vi "Get Information String.vi"(8 "error in (no error)":errorcluster caption="错误输入（无错误）", 11 "PCM PanelSplit.lvclass":refnum<class "PCM PanelSplit.lvclass">) -> (0 "error out":errorcluster caption="错误输出", 2 "Information String out":string, 3 "PCM PanelSplit out":refnum<class "PCM PanelSplit.lvclass"> caption="DNL_LabVIEW Object out")   [LabVIEW 2016, in "PCM PanelSplit.lvclass"]
uses:
  PCM PanelSplit.lvclass
  <vilib>/Analysis/4window.llb/windowTd.ctl
  <vilib>/Analysis/NI_AALPro.lvlib
panel:
  in  "window":T1 caption="窗" items=["Rectangle"=0, "Hanning"=1, "Hamming"=2, "Blackman-Harris"=3, "Exact Blackman"=4, "Blackman"=5, "Flat Top"=6, "4 Term B-Harris "=7, "7 Term B-Harris"=8, "Low Sidelobe"=9, "Blackman Nuttall"=11, "Triangle"=30, "Bartlett-Hanning"=31, "Bohman"=32, "Parzen"=33, "Welch"=34, "Kaiser"=60, "Dolph-Chebyshev"=61, "Gaussian"=62]
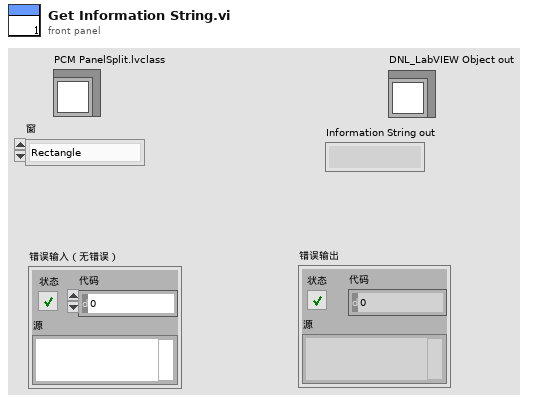
[diagram p1: front panel]
types:
  T1 = typedef "NI_AALPro.lvlib/windowTd.ctl" = u32
  T2 = typedef "PCM PanelSplit.lvclass/Display Config.ctl" = cluster{"Display Mode":T3, "ChTag[]":string[], "window":T1, "Range":T4}
  T3 = typedef "PCM PanelSplit.lvclass/Display Mode.ctl" = enum16{"时域", "频谱", "功率谱"}
  T4 = typedef "LVRangeTypeDef.ctl" = cluster{"Minimum":dbl, "Maximum":dbl, "Increment":dbl, "Minor Increment":dbl, "Start":dbl}
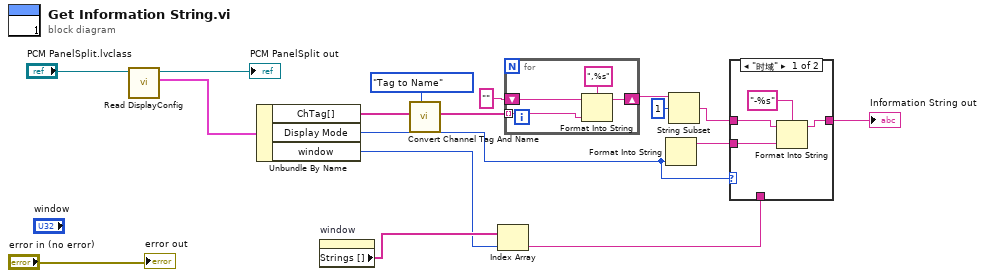
[diagram p0: block diagram]
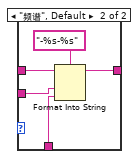
[diagram p2: hidden frame]
diagram:
  n1 = call "Read DisplayConfig.vi"("PCM PanelSplit 输入"="PCM PanelSplit.lvclass") -> ("Display Config"=w16:T2, "PCM PanelSplit 输出"=→"PCM PanelSplit out":refnum<class "PCM PanelSplit.lvclass">)  [unwired: 8 in, 1 out]
  n2 = Unbundle By Name(w16) -> ("ChTag[]"=w2:string[], "Display Mode"=w6:T3, "window"=w11:T1)
  n3 = property on="window" class="Ring (strict)"() -> ("Strings []"=w12:string[])  [unwired: 2 in, 2 out]
  n4 = call "Convert Channel Tag And Name.vi"("Direction"=enum16{"Tag to Name", "Name to Tag"}."Tag to Name", "String[] in"=w2) -> ("String[] out"=w1:string[])  [unwired: 8 in, 1 out]
  n5 = Index Array(array=w12, index=w11) -> (element=w10:string)
  n6 = for {
    tunnel: w1 -> [w18] mode=indexing
    shift-right: [w20] -> w15
    shift-left: "" -> [w19]
    n7 = Format Into String(format string=",%s" ("格式字符串"), initial string=w19, w18) -> (resulting string=w20:string)  [unwired: 1 in, 1 out]
  }
  n8 = Format Into String(w6) -> (resulting string=w13:string)  [unwired: 3 in, 1 out]
  n9 = String Subset(string=w15, offset (0)=1 ("偏移量(0)")) -> (substring=w14:string)  [unwired: 1 in]
  n10 = case shown="\"时域\"" w6 {
    tunnel: w14 -> [w25 w30]
    tunnel: w13 -> [w24 w28]
    tunnel: w10 -> [_ w27]
    tunnel: [w22 w26] -> w9
    frame "时域" {
      n11 = Format Into String(format string="-%s" ("格式字符串"), initial string=w25, w24) -> (resulting string=w22:string)  [unwired: 1 in, 1 out]
    }
    frame "频谱", Default {
      n12 = Format Into String(format string="-%s-%s" ("格式字符串"), initial string=w30, w28, w27) -> (resulting string=w26:string)  [unwired: 1 in, 1 out]
    }
  }
  "Information String out" <- w9
  "error out" <- "error in (no error)"
